vi "pathToString.vi"(8 "error in (no error)":errorcluster, 11 "PlayFile in":refnum<class "PlayFile.lvclass">) -> (0 "error out":errorcluster, 2 "pathString":string, 3 "PlayFile out":refnum<class "PlayFile.lvclass">)   [LabVIEW 2009, in "Tools.lvlib" / "Scripting.lvlib" / "PlayFile.lvclass"]
uses:
  PlayFile.lvclass
  PlayFile.lvclass/PlayFile.ctl
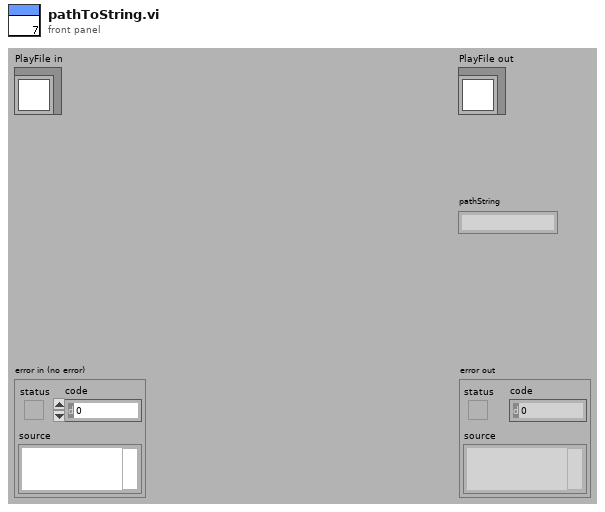
[diagram p1: front panel]
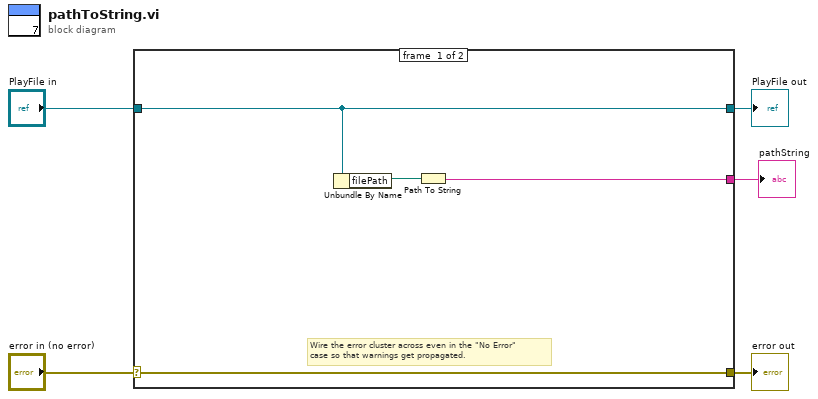
[diagram p0: block diagram]
diagram:
  n1 = case shown="No Error" "error in (no error)" {
    selector: "error in (no error)" -> [w9 w11]
    tunnel: [w9 w11] -> w4
    tunnel: [w7 w10] -> w2
    tunnel: "PlayFile in" -> [w7 w10]
    tunnel: [w8 _] -> w1
    frame #0 {
      # "Wire the error cluster across even in the \"No Error\"\ncase so that warnings get propagated."
      n2 = Unbundle By Name(w7) -> ("filePath"=w6:path)
      n3 = Path To String(path=w6) -> (string=w8:string)
    }
    frame #1 {
    }
  }
  "error out" <- w4
  "PlayFile out" <- w2
  "pathString" <- w1
